vi "Position Panel.vi"(0 "reference":refnum<vi>, 11 "error in (no error)":errorcluster) -> (4 "reference out":refnum<vi>, 15 "error out":errorcluster)   [LabVIEW 2015]
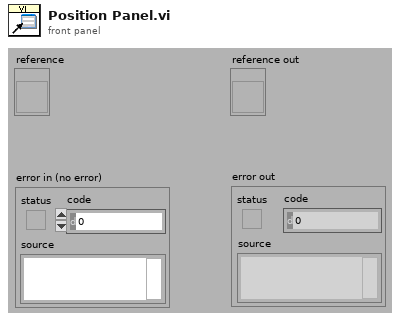
[diagram p1: front panel]
types:
  T1 = typedef "LVRectTypeDef.ctl" = cluster{"Left":i16, "Top":i16, "Right":i16, "Bottom":i16}
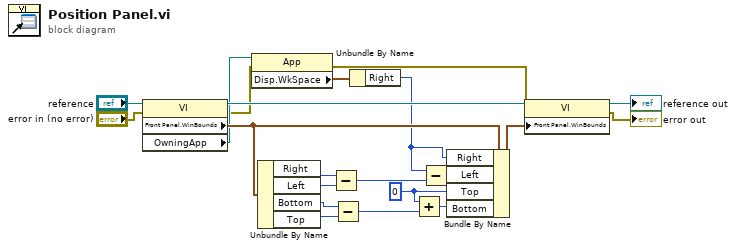
[diagram p0: block diagram]
diagram:
  w2 = i16 0
  n1 = property class="VI"(reference="reference", error in="error in (no error)") -> (reference out=w18:refnum<vi>, error out=w5:errorcluster, "Front Panel.WinBounds"=w15:T1, "OwningApp"=w8:refnum<vi>)
  n2 = property class="App"(reference=w8, error in=w5) -> (error out=w4:errorcluster, "Disp.WkSpace"=w7:T1)  [unwired: 1 out]
  n3 = Unbundle By Name(w15) -> ("Right"=w13:i16, "Left"=w14:i16, "Bottom"=w12:i16, "Top"=w11:i16)
  n4 = Subtract(x=w13, y=w14) -> (x-y=w10:i16)
  n5 = Subtract(x=w12, y=w11) -> (x-y=w3:i16)
  n6 = Unbundle By Name(w7) -> ("Right"=w6:i16)
  n7 = Add(x=w2, y=w3) -> (x+y=w1:i16)
  n8 = Subtract(x=w6, y=w10) -> (x-y=w9:i16)
  n9 = Bundle By Name(cluster=w15, "Right"=w6, "Left"=w9, "Top"=w2, "Bottom"=w1) -> (w19:T1)
  n10 = property class="VI"(reference=w18, error in=w4, "Front Panel.WinBounds"=w19) -> (reference out=→"reference out":refnum<vi>, error out=→"error out":errorcluster)
